vi "finishGoalKickEnemyPlayVSS.vi"(8 "error in (no error)":errorcluster, 10 "Game in":refnum<class "Game.lvclass">, 11 "GoalKickEnemyPlayVSS in":refnum<class "GoalKickEnemyPlayVSS.lvclass">) -> (0 "error out":errorcluster, 3 "GoalKickEnemyPlayVSS out":refnum<class "GoalKickEnemyPlayVSS.lvclass">)   [LabVIEW 2020, in "GoalKickEnemyPlayVSS.lvclass"]
uses:
  GoalKickEnemyPlayVSS.lvclass
  Game_class/Game.lvclass
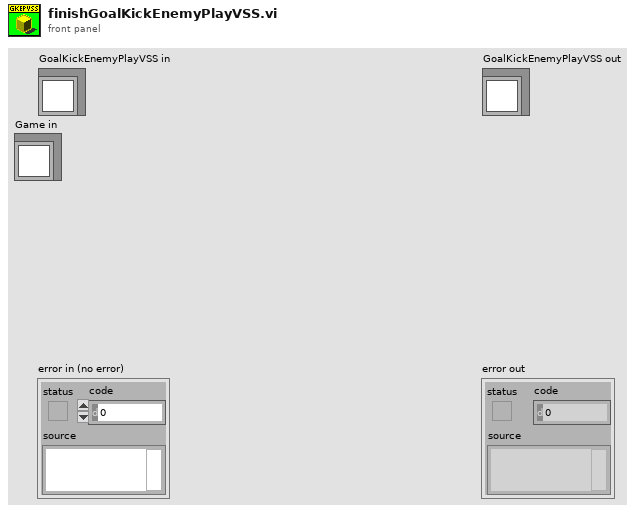
[diagram p1: front panel]
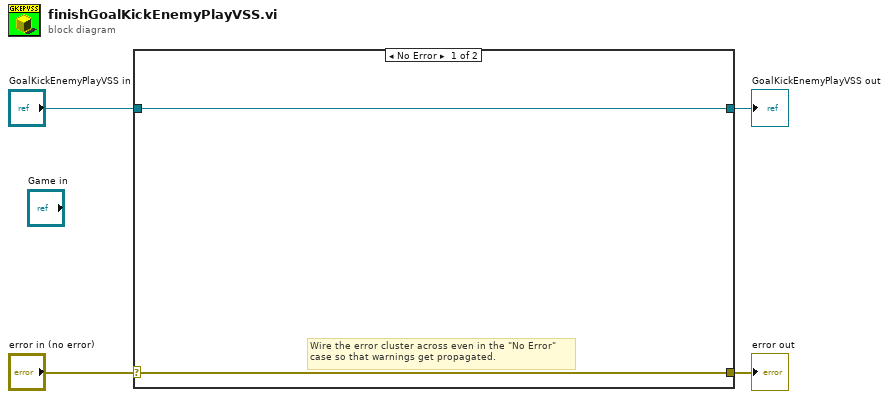
[diagram p0: block diagram]
diagram:
  n1 = case shown="No Error" "error in (no error)" {
    selector: "error in (no error)" -> [w5 w8]
    tunnel: [w5 w8] -> w3
    tunnel: [w6 w7] -> w1
    tunnel: "GoalKickEnemyPlayVSS in" -> [w6 w7]
    frame No Error {
      # "Wire the error cluster across even in the \"No Error\"\ncase so that warnings get propagated."
    }
    frame Error {
    }
  }
  "error out" <- w3
  "GoalKickEnemyPlayVSS out" <- w1
